vi "completeBroadcastStepMotorFrame.vi"(0 "HardPointActuator in":refnum<class "HPILC.lvclass">, 5 "FixedFrameBuilder":refnum<class "FixedFrameBuilder.lvclass">, 7 "WaitForTrigger":bool, 9 "TriggerIRQ":bool, 11 "error in (no error)":errorcluster) -> (4 "HardPointActuator out":refnum<class "HPILC.lvclass">, 6 "Frame":T1 {"Data" format="%02x"}, 15 "error out":errorcluster)   [LabVIEW 2015, in "RTHPILC.lvlib" / "HPILC.lvclass"]
uses:
  HPILC.lvclass
  Common_RT_Modbus/FixedFrameBuilder/FixedFrameBuilder.lvclass
  Common_RT_Modbus/DataTypes/Frame.ctl
  Common_RT_Modbus/RTModbus.lvlib
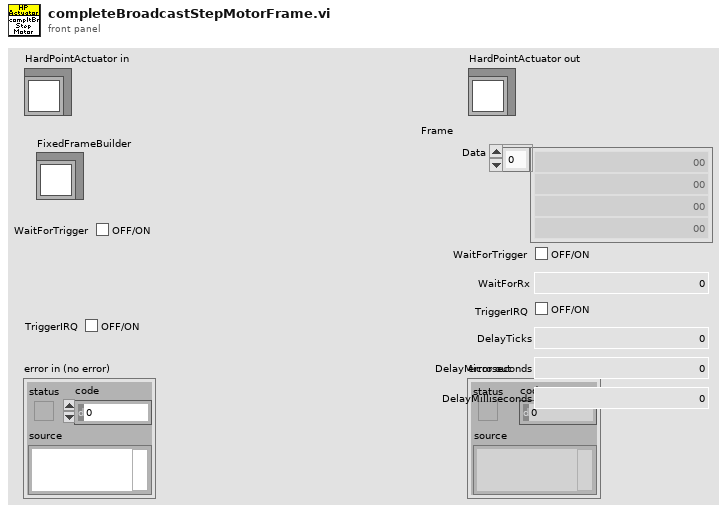
[diagram p1: front panel]
types:
  T1 = typedef "RTModbus.lvlib/Frame.ctl" = cluster{"Data":u8[], "WaitForTrigger":bool, "WaitForRx":u16, "TriggerIRQ":bool, "DelayTicks":u16, "DelayMicroseconds":u16, "DelayMilliseconds":u16}
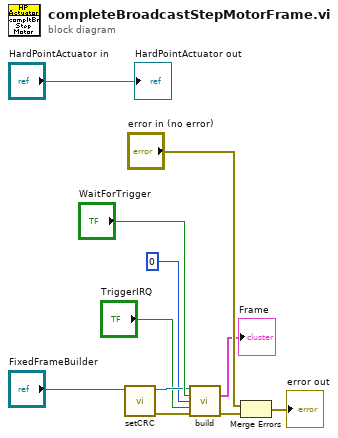
[diagram p0: block diagram]
diagram:
  n1 = call "setCRC.vi"("FixedFrameBuilder in"="FixedFrameBuilder") -> ("error out"=w3:errorcluster, "FixedFrameBuilder out"=w6:refnum<class "FixedFrameBuilder.lvclass">)  [unwired: 9 in]
  n2 = call "build.vi"("FixedFrameBuilder in"=w6, "WaitForTrigger"="WaitForTrigger", "WaitForRxTimeout"=u16 0, "TriggerIRQ"="TriggerIRQ", "error in (no error)"=w3) -> ("Frame"=→"Frame":T1, "error out"=w2:errorcluster)  [unwired: 8 in, 1 out]
  n3 = Merge Errors("error in (no error)", w2) -> (→"error out":errorcluster)
  "HardPointActuator out" <- "HardPointActuator in"
